vi "Configure Acquisition.vi"(8 "error in (no error)":errorcluster, 11 "Scope PXI Base CFG in":refnum<class "Scope PXI Base CFG.lvclass">) -> (0 "error out":errorcluster, 3 "Scope PXI Base CFG out":refnum<class "Scope PXI Base CFG.lvclass">)   [LabVIEW 2023, in "Scope PXI Base CFG.lvclass"]
uses:
  Scope PXI Base CFG.lvclass
  <instrlib>/niScope/Controls/niScope acquisition type.ctl
  Configuration/Configuration JSON/Configuration JSON Base/CFG JSON.lvclass/CFG JSON.ctl
  Scope PXI Base CFG.lvclass/Scope PXI Base CFG.ctl
  51f59c3a-b204-4edc-9e9c-c04e48498727.vi
  <vilib>/JDP Science/JSONtext/Find Item.vi
  <vilib>/JDP Science/JSONtext/Next JSON Value.vi
  <vilib>/JDP Science/JSONtext/String Subset.vi
  <vilib>/JDP Science/JSONtext/Parsing/Advance past next JSON Value (inlined COPY).vi
  <vilib>/JDP Science/JSONtext/Parsing/Advance past whitespace.vi
  <vilib>/JDP Science/JSONtext/Parsing/Advance past String.vi
  <vilib>/JDP Science/JSONtext/Parsing/Advance past Number.vi
  <vilib>/JDP Science/JSONtext/Parsing/Advance past Line Ending.vi
  <vilib>/JDP Science/JSONtext/Parsing/Parse Full Path or Item Name.vi
  <vilib>/JDP Science/JSONtext/Parsing/Advance past Array.vi
  <vilib>/JDP Science/JSONtext/Parsing/Advance past Object.vi
  <vilib>/JDP Science/JSONtext/support/Error Cluster From Code.vi
  <vilib>/JDP Science/JSONtext/Offset/Find Item Locations by Path.vi
  <vilib>/JDP Science/JSONtext/JSON text to Variant.vi
  <vilib>/Utility/error.llb/Error Cluster From Error Code.vi
  <vilib>/JDP Science/JSONtext/LVClass Serializer/JSONtext LVClass Serializer.lvclass
  <vilib>/ErrorRing/Error Ring.xnode
  Configuration/Configuration JSON/Configuration JSON Base/CFG JSON.lvclass
panel:
  out "Fetch Relative To":i32(ring)=388 items=["Start"=482, "Trigger"=483, "Pretrigger"=477, "Now"=481, "Read Pointer"=388]
  out "acquisition Type":T1 caption="Acquisition type (Normal)" items=["Normal"=0, "Flex Res"=1, "DDC"=3]
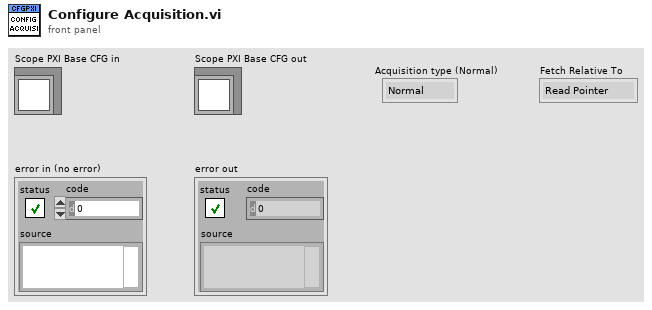
[diagram p1: front panel]
types:
  T1 = typedef "niScope acquisition type.ctl" = i32
  T2 = cluster{"Type":string, "Fetch Relative To":string}
  T3 = typedef "LVStringsAndValuesArrayTypeDef_I32.ctl" = cluster{"String":string, "Value":i32}[]
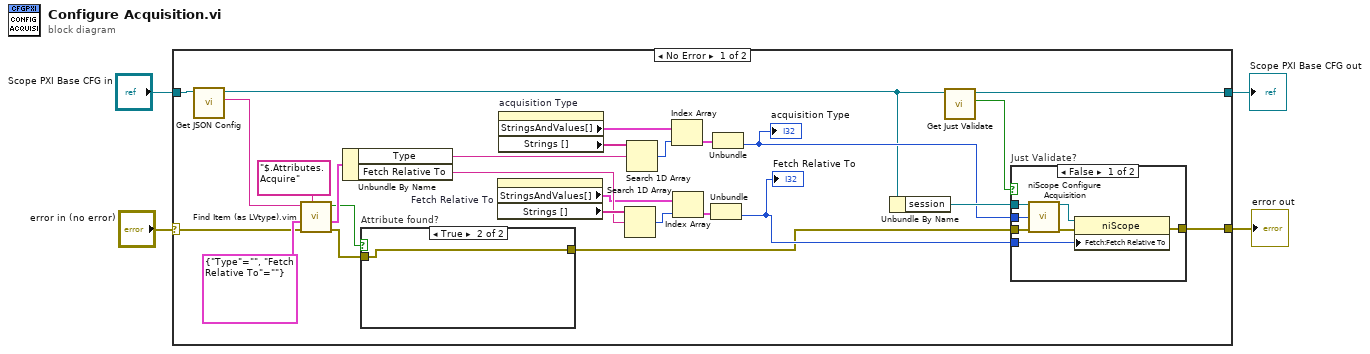
[diagram p0: block diagram]
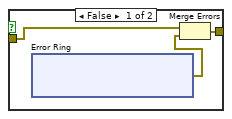
[diagram p3: hidden frame]
diagram:
  n1 = case shown="No Error" "error in (no error)" {
    selector: "error in (no error)" -> [w5 w49]
    tunnel: [w25 w49] -> w3
    tunnel: [w7 w48] -> w1
    tunnel: "Scope PXI Base CFG in" -> [w22 w48]
    frame No Error {
      n2 = call "Get JSON Config.vi"("CFG Base in"=w22) -> ("<JSON>Config>"=w20:string, "CFG Base out"=w21:refnum<class "Scope PXI Base CFG.lvclass">)  [unwired: 9 in]
      n3 = call "Find Item (as LVtype).vim"("$Path or Item Name"="$.Attributes.Acquire", "error in (no error)"=w5, "Data Type and Default Value"=T2 {"Type"="", "Fetch Relative To"=""}, "JSON"=w20) -> ("error out"=w9:errorcluster, "Data"=w18:T2, "Found"=w10:bool)  [unwired: 4 in, 1 out]
      n4 = Unbundle By Name(w18) -> ("Type"=w17:string, "Fetch Relative To"=w15:string)
      n5 = case "Attribute found?" shown="True" w10 {
        tunnel: w9 -> [w41 w47]
        tunnel: [w39 w47] -> w8
        frame False {
          n6 = xnode "Error Ring"() -> ("error out"=w40:errorcluster)
          n7 = Merge Errors(w41, w40) -> (w39:errorcluster)
        }
        frame True {
        }
      }
      n8 = property on="Fetch Relative To" class="Ring (strict)"() -> ("StringsAndValues[]"=w13:T3, "Strings []"=w16:string[])  [unwired: 2 in, 2 out]
      n9 = property on="acquisition Type" class="Ring (strict)"() -> ("StringsAndValues[]"=w28:T3, "Strings []"=w29:string[])  [unwired: 2 in, 2 out]
      n10 = Search 1D Array(1D array=w16, element=w15) -> (index of element=w14:i32)  [unwired: 1 in]
      n11 = Search 1D Array(1D array=w29, element=w17) -> (index of element=w27:i32)  [unwired: 1 in]
      n12 = Index Array(array=w28, index=w27) -> (element=w26:cluster{"String":string, "Value":i32})
      n13 = Index Array(array=w13, index=w14) -> (element=w12:cluster{"String":string, "Value":i32})
      n14 = Unbundle(w12) -> ("Value"=w11:i32)  [unwired: 1 out]
      "Fetch Relative To" <- w11
      n15 = Unbundle(w26) -> ("Value"=w23:i32)  [unwired: 1 out]
      "acquisition Type" <- w23
      n16 = Unbundle By Name(w21) -> ("session"=w24:refnum<k15>)
      n17 = call "Get Just Validate.vi"("CFG JSON Base in"=w21) -> ("Just Validate"=w6:bool, "CFG JSON Base out"=w7:refnum<class "Scope PXI Base CFG.lvclass">)  [unwired: 9 in]
      n18 = case "Just Validate?" shown="False" w6 {
        tunnel: [w37 w38] -> w25
        tunnel: w24 -> [w36 _]
        tunnel: w23 -> [w35 _]
        tunnel: w11 -> [w34 _]
        tunnel: w8 -> [w31 w38]
        frame False {
          n19 = call <instrlib>:"niScope Configure Acquisition.vi"("instrument handle"=w36, "acquisition Type"=w35, "error in"=w31) -> ("instrument handle out"=w32:refnum<k15>, "error out"=w33:errorcluster)  [unwired: 11 in]
          n20 = property class="niScope"(reference=w32, error in=w33, "Fetch:Fetch Relative To"=w34) -> (error out=w37:errorcluster)  [unwired: 1 out]
        }
        frame True {
        }
      }
    }
    frame Error {
    }
  }
  "error out" <- w3
  "Scope PXI Base CFG out" <- w1
